vi "Copy Image (Greyscale with Mask).vi"(8 "error in (no error)":errorcluster, 9 "Greyscale Image Mask":T1, 10 "Greyscale Image Destination":T1, 11 "Greyscale Image Source":T1) -> (0 "error out":errorcluster, 3 "Greyscale Image Destination (duplicate)":T1)   [LabVIEW 2020, in "image.lvlib"]
uses:
  image.lvlib
  Greyscale Image.ctl
  1519c485-f8d8-4564-b4f6-4c035770646f.vi
  common/Module Path.vi
  <vilib>/Utility/error.llb/Error Cluster From Error Code.vi
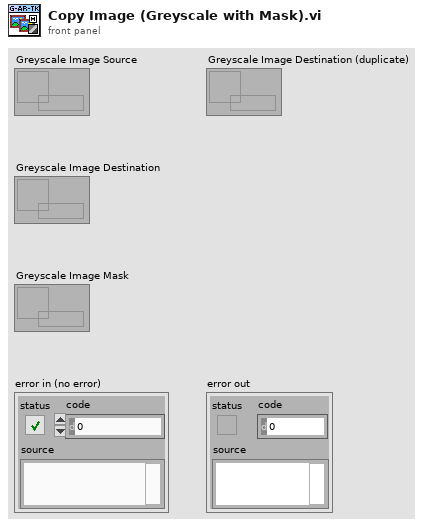
[diagram p1: front panel]
types:
  T1 = typedef "image.lvlib/Greyscale Image.ctl" = refnum<data-value>
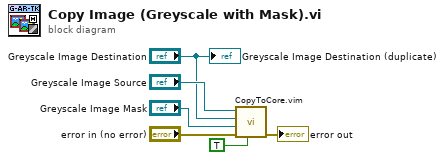
[diagram p0: block diagram]
diagram:
  n1 = call "CopyToCore.vim"("Has Mask"=TRUE, "error in (no error)"="error in (no error)", "Mask"="Greyscale Image Mask", "Dst"="Greyscale Image Destination", "Src"="Greyscale Image Source") -> ("error out"=→"error out":errorcluster)  [unwired: 6 in]
  "Greyscale Image Destination (duplicate)" <- "Greyscale Image Destination"
